vi "Discover Power Supply Model.vi"(10 "Model In":string) -> (2 "selection":bool)   [LabVIEW 2018]
panel:
  out "size(s)":i32
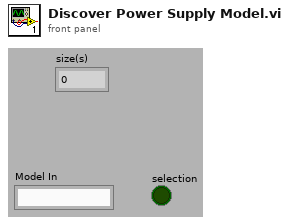
[diagram p1: front panel]
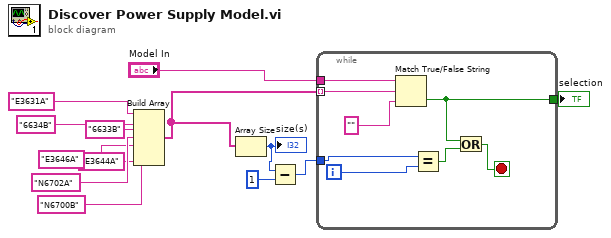
[diagram p0: block diagram]
diagram:
  n1 = Build Array("E3631A" ("true string"), "6634B" ("true string"), "6633B" ("element"), "N6702A" ("element"), "E3646A" ("element"), "N6700B" ("element"), "E3644A" ("element")) -> (w9:string[])
  n2 = Array Size(array=w9) -> (size(s)=w8:i32)
  "size(s)" <- w8
  n3 = Subtract(x=w8, y=1) -> (x-y=w6:i32)
  n4 = while {
    tunnel: w9 -> [w20] mode=indexing
    tunnel: "Model In" -> [w19]
    tunnel: [w18] -> w10
    tunnel: w6 -> [w14]
    i -> [w15]
    stop <- w17 stop-if-true
    n5 = Match True/False String(2:"" ("false string"), 3:w20, 4:w19) -> (0:w18:bool)  [unwired: 1 out]
    n6 = Equal?(x=w14, y=w15) -> (x = y?=w16:bool)
    n7 = Or(x=w18, y=w16) -> (x .or. y?=w17:bool)
  }
  "selection" <- w10
